vi "Dashboard Main.vi"() -> ()   [LabVIEW 2013]
uses:
  <vilib>/event_ctls.llb/eventvkey.ctl
  <vilib>/Rock Robotics/WPI/Dashboard/WPI_DashboardLogging Global.vi
  <vilib>/Utility/config.llb/Write Key (String).vi
  <vilib>/Utility/config.llb/Write Key (I32).vi
  <vilib>/Utility/config.llb/NI_LVConfig.lvlib
panel:
  out "Image Message":string="Timeout in Camera Communications"
  in  "Rec Mode":enum32{"Stop", "Record", "Playback"}(radio)
  in  "Dashboard Tab":T1(tab)
  out "Encoder Rate":dbl
  out "Encoder Count":dbl
  in  "Camera Settings":T2={"Frame Rate"=30, "Compression"=30, "Size"=1} {"Frame Rate" scale=1.0..30.0; "Size" items=["640x480", "320x240", "160x120"]}
  out "MotorSliders R":cluster{"MotorSlide1":dbl, "MotorSlide2":dbl} {"MotorSlide2" scale=-1.0..1.0 scale format="%#_2e"; "MotorSlide1" scale=-1.0..1.0 scale format="%#_2e"}
  out "MotorChart R":cluster{"Numeric":dbl, "Numeric":dbl}(graph)
  out "MotorSliders L":T3 {"MotorSlide4 2" scale=0.0..14.0 scale format="%#_2e"; "MotorSlide2" scale=-1.0..1.0 scale format="%#_2e"; "MotorSlide1" scale=-1.0..1.0 scale format="%#_2e"}
  out "MotorChart L":T4(graph)
  out "JS1 Z":dbl(slide) scale=-1.0..1.0 scale format="%#_2e"
  out "Joystick 1":cluster{"X":dbl, "Y":dbl}[](graph)
  out "JS Buttons 1":T5
  out "JS2 Z":dbl(slide) scale=-1.0..1.0 scale format="%#_2e"
  out "Joystick 2":cluster{"X":dbl, "Y":dbl}[](graph)
  out "JS Buttons 2":T5
  out "Mode":T6(ring)=enum."Auto Disabled"
  out "Camera IP":string
  in  "DB Camera Config":bool
  out "fps":dbl format="%#.1g"
  out "Mbps":dbl format="%#.1g"
  out "Mbps 2":bool
  out "LED 1":bool
  in  "Slider 1":dbl(slide) scale=0.0..100.0
  in  "Test Jag Num":u8
  in  "Test Jag Out":dbl min=-1.0 max=1.0
  in  "Checkbox 2":bool
  in  "Checkbox 1":bool
  in  "Test Slider":dbl(slide) scale=0.0..100.0 scale format="%#_3g"
  in  "On/Off":bool caption="Solenoid"
  in  "Test Name":u16(ring) items=["Select the test to run...", "Example Test", "-------------------------------", "List of tests is built in robot code.", "Replace with your own automated tests.", "Jag Test"]
  in  "Test Tree":string(tree)
  in  "Motor":cluster{"Value":dbl, "Enable":bool} {"Value" scale=-1.0..1.0 scale format="%#_3g"}
  out "Progress":T7 {"Test Progress" scale=0.0..100.0}
  in  "Rev/Fwd":cluster{"Forward":bool, "Reverse":bool}
  in  "Test Ring":u16(ring) items=["Auto", "Fixed indoor", "Fixed outdoor 1", "Fixed outdoor 2", "Fixed fluorescent 1", "Fixed fluorescent 2", "Hold current"]
  in  "Listbox":i32(listbox)
  out "Tree":string(tree)
  out "Camera Image":T8(plugin-control)
  in  "Enable":bool
  # "Left"
  # "Front"
  # "Right"
  # "Battery"
  # "Customize by placing controls and indicators here and name to\nmatch Dashboard Variables on robot."
  # "This tab is a great place for autonomous settings and validation.\nCustomize by placing controls and indicators here and name to\nmatch Dashboard Variables on robot."
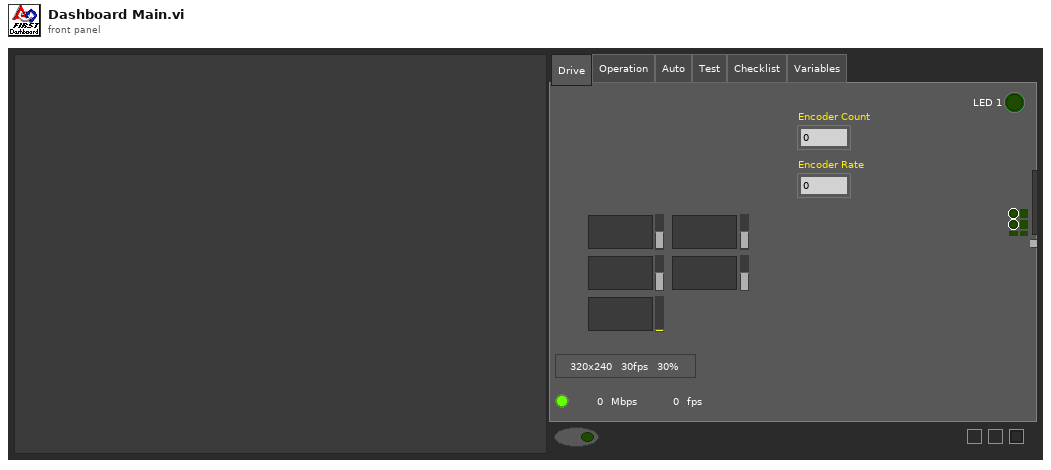
[diagram p1: front panel]
types:
  T1 = enum32{"Drive", "Operation", "Auto", "Test", "Checklist", "Variables"}
  T2 = cluster{"Frame Rate":i32, "Compression":i32, "Size":u16}
  T3 = cluster{"MotorSlide1":dbl, "MotorSlide2":dbl, "MotorSlide4 2":dbl}
  T4 = cluster{"Numeric":dbl, "Numeric":dbl, "Battery":sgl}
  T5 = cluster{bool, bool, bool, bool, bool, bool, bool, bool, bool, bool, bool, bool}
  T6 = enum8{"Tele-Op Disabled", "Tele-Op Enabled", "Auto Disabled", "Auto Enabled", "Test Disabled", "Test Enabled", ""}
  T7 = cluster{"Test Progress":u8, "Test Progress Text":string}
  T8 = typedef "IMAQ Image.ctl" = refnum<image>
  T9 = typedef "Image Type" = u32
  T10 = cluster{"Digital Inputs":bool[], "Digital Outputs":bool[]}
  T11 = cluster{"Competition mode":bool, "Robot Link":bool, "Autonomous":bool, "Enabled":bool, "E-Stop":bool, "Simulated":bool, "TestMode":bool, "Docked Window":bool}
  T12 = cluster{"Boolean Array[0]":bool, "Boolean Array[1]":bool, "Boolean Array[2]":bool, "Boolean Array[3]":bool, "Boolean Array[4]":bool, "Boolean Array[5]":bool, "Boolean Array[6]":bool, "Boolean Array[7]":bool, "Boolean Array[8]":bool, "Boolean Array[9]":bool, "Boolean Array[10]":bool, "Boolean Array[11]":bool}
  T13 = typedef "NI_LVConfig.lvlib/Config Data RefNum.ctl" = refnum<k1>
  T14 = typedef "eventvkey.ctl" = enum16{"ASCII", "Enter", "Return", "Shift", "Ctrl", "Alt", "Cmd", "Opt", "Caps", "NumLock", "Clear", "Break", "Up", "Down", "Left", "Right", "Insert", "Delete", "Home", "End", "PageUp", "PageDown", "Escape", "Help", "Pause", "ScrollLock", "F1", "F2", "F3", "F4", "F5", "F6", "F7", "F8", "F9", "F10", "F11", "F12", "F13", "F14", "F15", "F16", "F17", "F18", "F19", "F20", "F21", "F22", "F23", "F24", "Play", "VolumeUp", "VolumeDown", "Mute", "Two Byte Char"}
  T15 = cluster{"Image Size":bool, "Image Type":bool, "Pixel Value":bool, "ROI Information":bool, "Zoom Factor":bool}
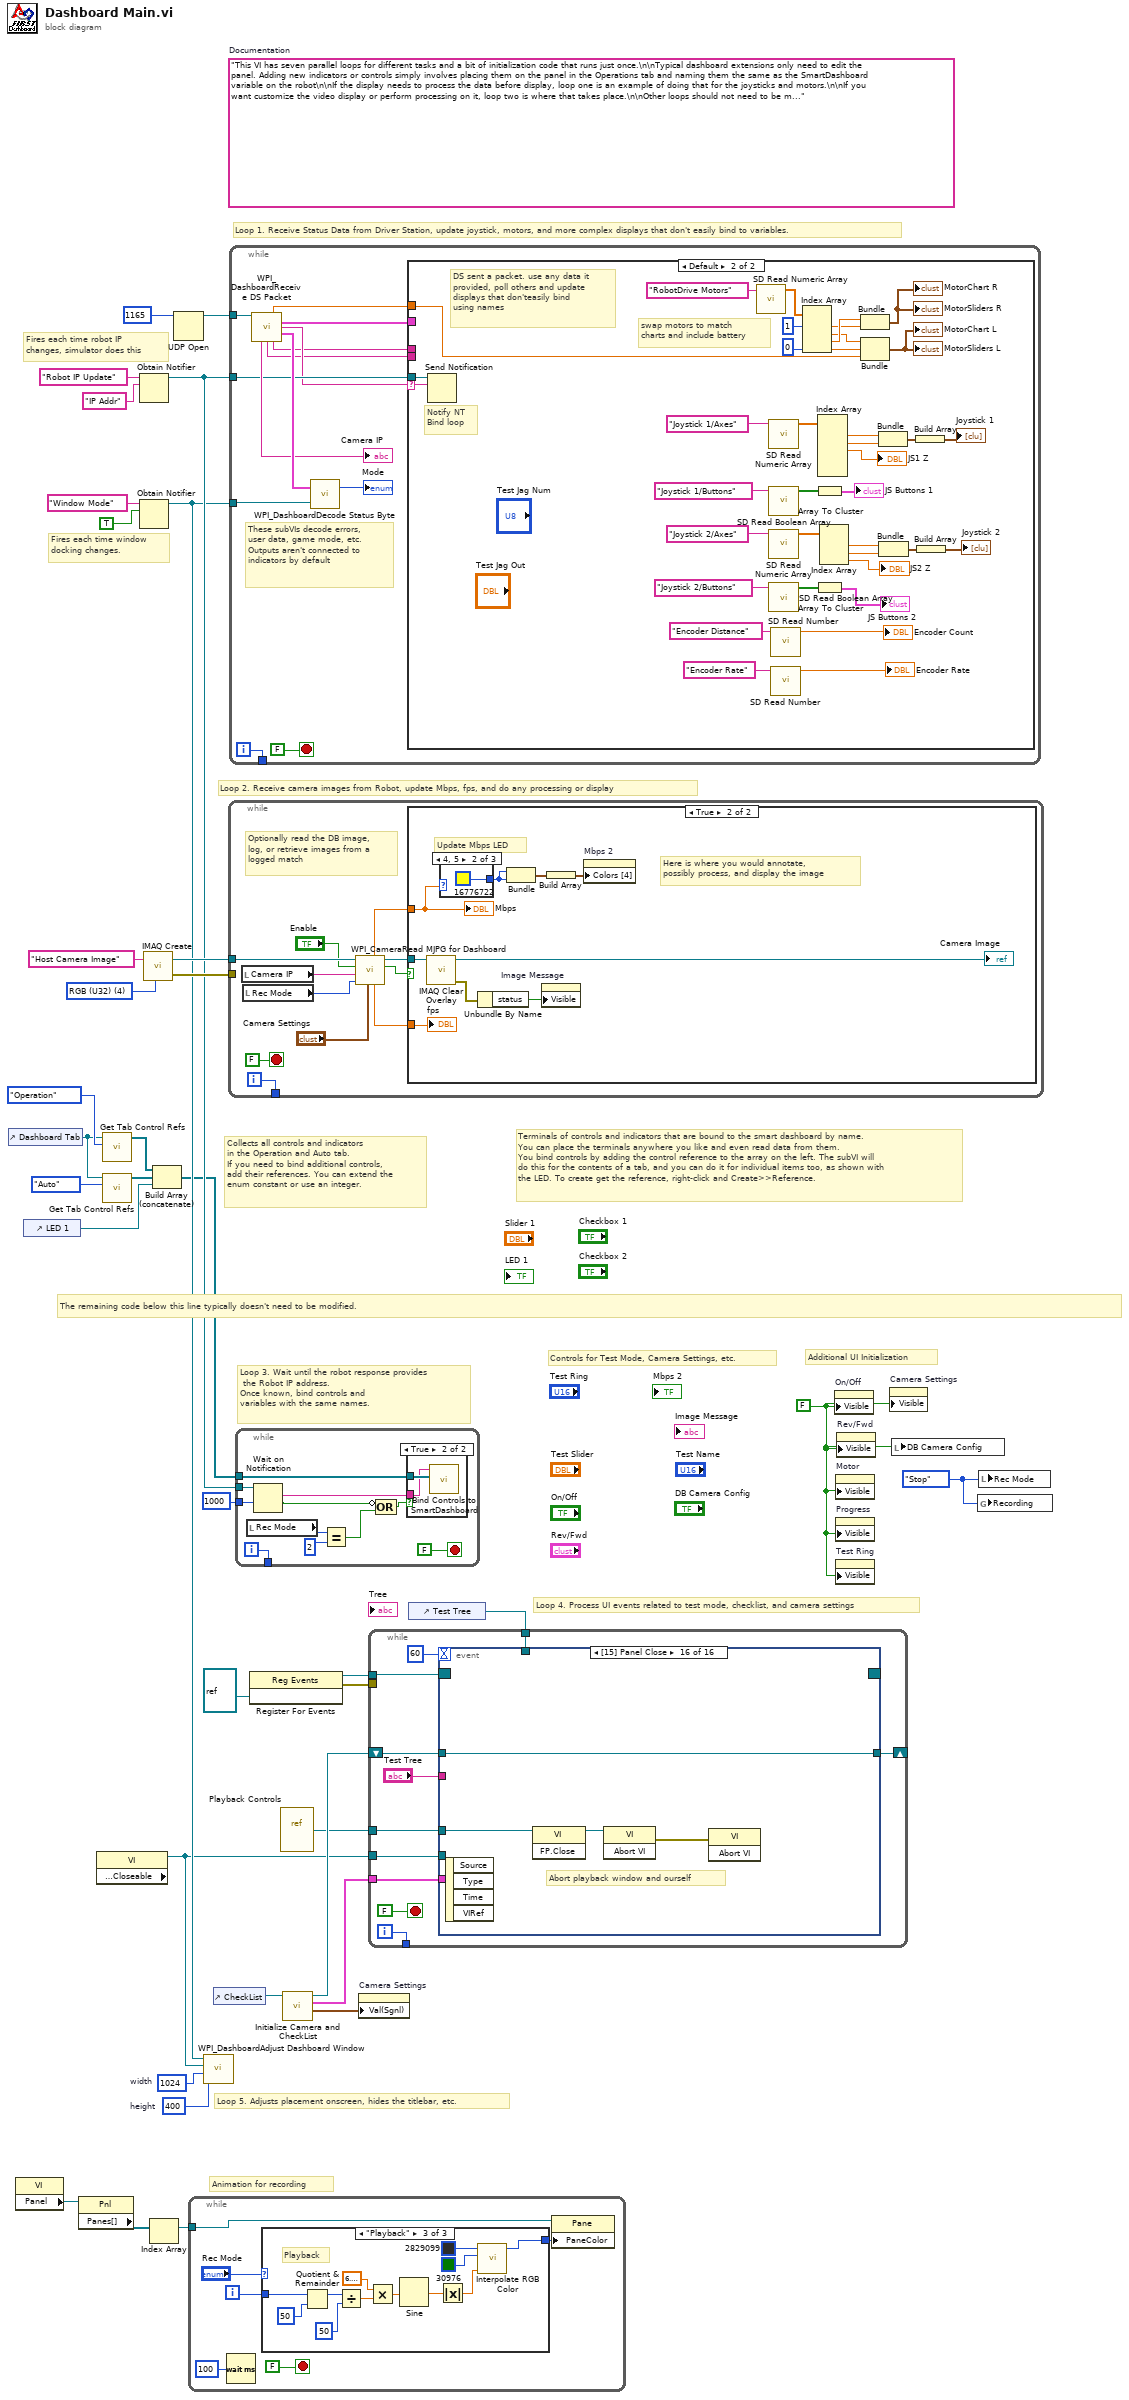
[diagram p0: block diagram]
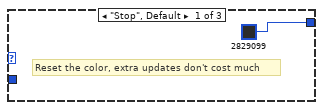
[diagram p2: hidden frame]
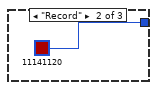
[diagram p3: hidden frame]
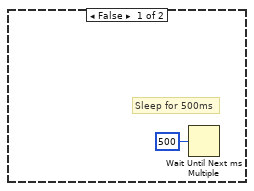
[diagram p5: hidden frame]
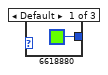
[diagram p6: hidden frame]
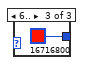
[diagram p7: hidden frame]
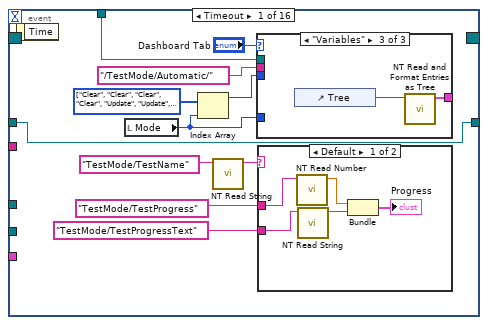
[diagram p8: hidden frame]
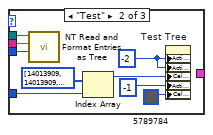
[diagram p10: hidden frame]
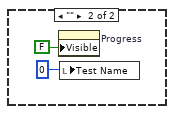
[diagram p11: hidden frame]
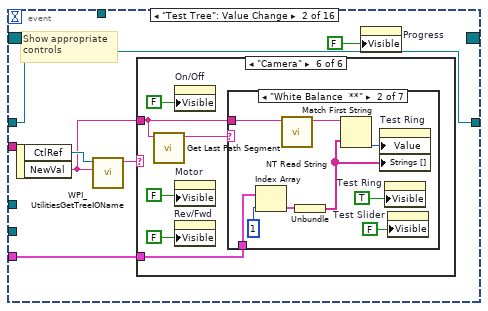
[diagram p12: hidden frame]
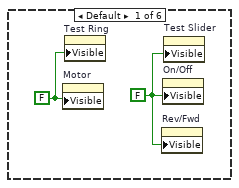
[diagram p13: hidden frame]
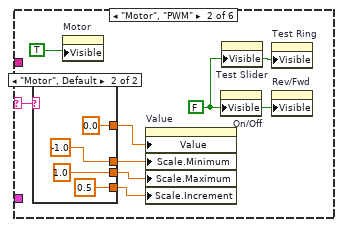
[diagram p14: hidden frame]
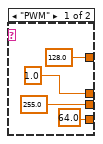
[diagram p15: hidden frame]
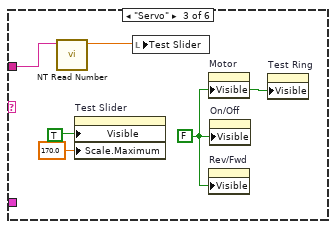
[diagram p16: hidden frame]
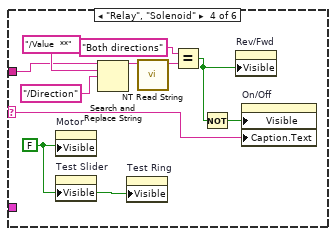
[diagram p17: hidden frame]
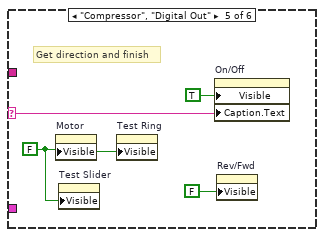
[diagram p18: hidden frame]
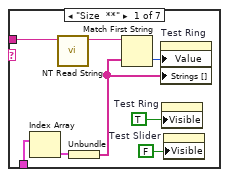
[diagram p19: hidden frame]
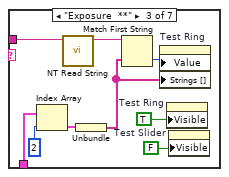
[diagram p20: hidden frame]
diagram:
  w8 = enum32{"Stop", "Record", "Playback"}."Stop" ("Rec Mode")
  w11 = 400  # height
  w12 = 1024  # width
  w25 = FALSE ("Visible")
  (unwired) "This VI has seven parallel loops for different tasks and a bit of initialization code that runs just once.\n\nTypical dashboard extensions only need to edit the panel. Adding new indicators or controls simply involves placing them on the panel in the Operations tab and naming them the same as the SmartDashboard variable on the robot\n\nIf the display needs to process the data before display, loop one is an example of doing that for the joysticks and motors.\n\nIf you want customize the video display or perform processing on it, loop two is where that takes place.\n\nOther loops should not need to be modified. They are pretty standard, and document the task they perform."  # Documentation
  w35 = T9 4 items=["Grayscale (U8)", "Grayscale (I16)", "Grayscale (SGL)", "Complex (CSG)", "RGB (U32)", "HSL (U32)", "RGB (U64)"] ("Image Type")
  # "Controls for Test Mode, Camera Settings, etc."
  # "Additional UI Initialization"
  # "Animation for recording"
  # "Fires each time robot IP\nchanges, simulator does this"
  # "Fires each time window\ndocking changes."
  # "Collects all controls and indicators\nin the Operation and Auto tab.\nIf you need to bind additional controls,\nadd their references. You can extend the\nenum constant or use an integer."
  # "The remaining code below this line typically doesn't need to be modified."
  # "Loop 4. Process UI events related to test mode, checklist, and camera settings"
  # "Terminals of controls and indicators that are bound to the smart dashboard by name.\nYou can place the terminals anywhere you like and even read data from them.\nYou bind controls by adding the control reference to the array on the left. The subVI will\ndo this for the contents of a tab, and you can do it for individual items too, as shown with\nthe LED. To create get the reference, right-click and Create>>Reference."
  # "Loop 3. Wait until the robot response provides\n the Robot IP address.\nOnce known, bind controls and\nvariables with the same names."
  # "Loop 5. Adjusts placement onscreen, hides the titlebar, etc."
  # "Loop 1. Receive Status Data from Driver Station, update joystick, motors, and more complex displays that don't easily bind to variables."
  # "Loop 2. Receive camera images from Robot, update Mbps, fps, and do any processing or display"
  n1 = control-ref of="Dashboard Tab"() -> (w6:refnum<vi>)
  n2 = property class="VI"() -> ("Panel"=w19:refnum<vi>)  [unwired: 2 in, 2 out]
  n3 = control-ref of="LED 1"() -> (w1:refnum<vi>)
  n4 = property class="Pnl"(reference=w19) -> ("Panes[]"=w20:refnum<vi>[])  [unwired: 1 in, 2 out]
  n5 = property class="VI" props=["Front Panel.Closeable"]() -> (reference out=w7:refnum<vi>)  [unwired: 2 in, 2 out]
  n6 = call <vilib>:"Get Tab Control Refs.vi"("Page Index"=T1."Operation" ("Dashboard Tab"), "TabControl in"=w6) -> ("ControlsOnPage"=w4:refnum<vi>[])  [unwired: 9 in]
  n7 = call <vilib>:"Get Tab Control Refs.vi"("Page Index"=T1."Auto" ("Dashboard Tab"), "TabControl in"=w6) -> ("ControlsOnPage"=w5:refnum<vi>[])  [unwired: 9 in]
  n8 = Obtain Notifier(name (unnamed)="Robot IP Update", notification data type="IP Addr" ("name (unnamed)")) -> (notifier out=w29:refnum<notifier>)  [unwired: 2 in, 2 out]
  n9 = Obtain Notifier(name (unnamed)="Window Mode", notification data type=TRUE) -> (notifier out=w10:refnum<notifier>)  [unwired: 2 in, 2 out]
  n10 = call "IMAQ Create"("Image Name"="Host Camera Image", "Image Type"=w35) -> ("New Image"=w33:T8, "error out"=w32:errorcluster)  [unwired: 2 in, 1 out]
  n11 = Index Array(array=w20) -> (element=w18:refnum<vi>)  [unwired: 1 in]
  n12 = Build Array (concatenate)(w4, w5, w1) -> (w3:refnum<vi>[])
  n13 = UDP Open(11:u16 1165 ("port")) -> (port=w36:refnum<k16>)  [unwired: 2 in, 4 out]
  n14 = while {
    tunnel: w18 -> [w39]
    i -> [w42]
    stop <- FALSE stop-if-true
    n15 = Wait (ms)(milliseconds to wait=u32 100) -> ()  [unwired: 1 out]
    n16 = case shown="\"Playback\"" "Rec Mode" {
      tunnel: w42 -> [_ _ w57]
      tunnel: [u32 2829099 ("Base Color") u32 11141120 ("Target Color") w46] -> w38
      frame "Stop", Default {
        # "Reset the color, extra updates don't cost much"
      }
      frame "Record" {
      }
      frame "Playback" {
        # "Playback"
        n17 = Quotient & Remainder(x=w57, y=u32 50 ("milliseconds to wait")) -> (x-y*floor(x/y)=w53:u32)  [unwired: 1 out]
        n18 = Divide(x=w53, y=u32 50 ("milliseconds to wait")) -> (x/y=w50:dbl)
        n19 = Multiply(x=6.283185307179586, y=w50) -> (x*y=w55:dbl)
        n20 = Sine(x=w55) -> (sin(x)=w54:dbl)
        n21 = Absolute Value(x=w54) -> (abs(x)=w47:dbl)
        n22 = call "Interpolate RGB Color.vi"("Proportion"=w47, "Target Color"=u32 30976, "Base Color"=u32 2829099) -> ("Result Color"=w46:u32)  [unwired: 8 in]
      }
    }
    n23 = property class="Pane"(reference=w39, "PaneColor"=w38) -> ()  [unwired: 1 in, 2 out]
  }
  n24 = call <vilib>:"WPI_DashboardAdjust Dashboard Window.vi"("height"=w11, "width"=w12, "reference in"=w7, "Notifier in"=w10) -> ()  [unwired: 8 in]
  n25 = control-ref of="CheckList"() -> (w9:refnum<vi>)
  n26 = while {
    tunnel: w33 -> [w66]
    tunnel: w32 -> [_]
    tunnel: [w67] -> _
    i -> [w67]
    stop <- FALSE stop-if-true
    # "Optionally read the DB image,\nlog, or retrieve images from a\nlogged match"
    n27 = local read "Camera IP"() -> (w59:string)
    n28 = local read "Rec Mode"() -> (w58:enum32{"Stop", "Record", "Playback"})
    n29 = call <vilib>:"WPI_CameraRead MJPG for Dashboard.vi"("Camera Settings"="Camera Settings", "Rec Mode"=w58, "Camera IP"=w59, "Enable"="Enable", "Refnum in"=w66) -> ("Active"=w63:bool, "Refnum out"=w65:T8, "FPS"=w62:dbl, "Bandwidth (Mbps)"=w61:dbl)  [unwired: 3 in]
    n30 = case shown="True" w63 {
      tunnel: w65 -> [_ w73]
      tunnel: w61 -> [_ w72]
      tunnel: w62 -> [_ w70]
      frame False {
        # "Sleep for 500ms"
        n31 = Wait Until Next ms Multiple(millisecond multiple=u32 500) -> ()  [unwired: 1 out]
      }
      frame True {
        # "Here is where you would annotate,\npossibly process, and display the image"
        # "Update Mbps LED"
        n32 = call "IMAQ Clear Overlay"("Image"=w73) -> ("error out"=w77:errorcluster, "Image Out"=→"Camera Image":T8)  [unwired: 2 in, 7 out]
        n33 = case shown="4, 5" w72 {
          tunnel: [u32 6618880 ("Color Box") u32 16776722 ("Color Box") u32 16716800 ("Color Box")] -> w74
          frame Default {
          }
          frame 4, 5 {
          }
          frame 6.. {
          }
        }
        n34 = Unbundle By Name(w77) -> ("status"=w78:bool)
        n35 = Bundle("Color Box"=w74, "Color Box"=w74) -> (w76:cluster{"Color Box":u32, "Color Box":u32})  [unwired: 1 out]
        n36 = property on="Image Message" class="Str"("Visible"=w78) -> ()  [unwired: 2 in, 2 out]
        n37 = Build Array(w76) -> (w75:cluster{"Color Box":u32, "Color Box":u32}[])
        n38 = property on="Mbps 2" class="Bool (strict)"("Colors [4]"=w75) -> ()  [unwired: 2 in, 2 out]
        "Mbps" <- w72
        "fps" <- w70
      }
    }
  }
  n39 = while {
    tunnel: w36 -> [w92]
    tunnel: w29 -> [w87]
    tunnel: w10 -> [w91]
    tunnel: [w88] -> _
    i -> [w88]
    stop <- FALSE stop-if-true
    # "These subVIs decode errors, user data, game mode, etc.\nOutputs aren't connected to indicators by default"
    n40 = call <vilib>:"WPI_DashboardReceive DS Packet.vi"("Recv Socket"=w92) -> ("Battery"=w82:sgl, "Driver Station"=w83:T10, "Robot IP Address"=w86:string, "Status"=w93:T11, "Camera IP Address"=→"Camera IP":string, "Low Priority User Data"=w85:string, "High Priority User Data"=w84:string)  [unwired: 1 in, 7 out]
    n41 = call <vilib>:"WPI_DashboardDecode Status Byte.vi"("Window Mode Notifier"=w91, "Status"=w93) -> ("Mode"=→"Mode":T6)  [unwired: 1 out]
    n42 = case shown="Default" w86 {
      selector: w86 -> [_ w109]
      tunnel: w87 -> [_ w110]
      tunnel: w85 -> [_ _]
      tunnel: w84 -> [_ _]
      tunnel: w83 -> [_ _]
      tunnel: w82 -> [_ w108]
      frame "0.0.0.0" {
        # "DS not sending packets, or no robot exists yet.\nDon't poll the variables"
      }
      frame Default {
        # "Notify NT\nBind loop"
        # "DS sent a packet. use any data it\nprovided, poll others and update\ndisplays that don'teasily bind\nusing names"
        # "swap motors to match\ncharts and include battery"
        n43 = Send Notification(notification=w109, notifier=w110) -> ()  [unwired: 1 in, 2 out]
        n44 = call <vilib>:"SD Read Numeric Array.vi"("Name"="RobotDrive Motors") -> ("Numeric Array"=w107:dbl[])  [unwired: 8 in, 2 out]
        n45 = call <vilib>:"SD Read Numeric Array.vi"("Name"="Joystick 1/Axes") -> ("Numeric Array"=w126:dbl[])  [unwired: 8 in, 2 out]
        n46 = call <vilib>:"SD Read Boolean Array.vi"("Name"="Joystick 1/Buttons") -> ("Boolean Array"=w128:bool[])  [unwired: 8 in, 2 out]
        n47 = call <vilib>:"SD Read Numeric Array.vi"("Name"="Joystick 2/Axes") -> ("Numeric Array"=w120:dbl[])  [unwired: 8 in, 2 out]
        n48 = call <vilib>:"SD Read Boolean Array.vi"("Name"="Joystick 2/Buttons") -> ("Boolean Array"=w119:bool[])  [unwired: 8 in, 2 out]
        n49 = call <vilib>:"SD Read Number.vi"("Name"="Encoder Distance") -> ("Numeric"=→"Encoder Count":dbl)  [unwired: 8 in, 2 out]
        n50 = call <vilib>:"SD Read Number.vi"("Name"="Encoder Rate") -> ("Numeric"=→"Encoder Rate":dbl)  [unwired: 8 in, 2 out]
        n51 = Index Array(array=w107, index #1=1, index #4=0) -> (element #1=w103:dbl, element #2=w102:dbl, element #3=w104:dbl, element #4=w99:dbl)  [unwired: 2 in]
        n52 = Array To Cluster(array=w128) -> (cluster=→"JS Buttons 1":T12)
        n53 = Array To Cluster(array=w119) -> (cluster=→"JS Buttons 2":T12)
        n54 = Index Array(array=w126) -> (element #1=w123:dbl, element #2=w124:dbl, element #3=→"JS1 Z":dbl)  [unwired: 6 in, 3 out]
        n55 = Index Array(array=w120) -> (element #1=w115:dbl, element #2=w114:dbl, element #3=→"JS2 Z":dbl)  [unwired: 3 in]
        n56 = Bundle("Numeric"=w104, "Numeric"=w103) -> (→"MotorChart R" →"MotorSliders R":cluster{"Numeric":dbl, "Numeric":dbl})  [unwired: 1 in]
        n57 = Bundle("Numeric"=w102, "Numeric"=w99, "Battery"=w108) -> (→"MotorChart L" →"MotorSliders L":T4)  [unwired: 1 in]
        n58 = Bundle("Numeric"=w123, "Numeric"=w124) -> (w122:cluster{"Numeric":dbl, "Numeric":dbl})  [unwired: 1 in]
        n59 = Bundle("Numeric"=w115, "Numeric"=w114) -> (w116:cluster{"Numeric":dbl, "Numeric":dbl})  [unwired: 1 in]
        n60 = Build Array(w122) -> (→"Joystick 1":cluster{"Numeric":dbl, "Numeric":dbl}[])
        n61 = Build Array(w116) -> (→"Joystick 2":cluster{"Numeric":dbl, "Numeric":dbl}[])
      }
    }
  }
  n62 = while {
    tunnel: w3 -> [w142]
    tunnel: w29 -> [w140]
    tunnel: [w138] -> _
    tunnel: u32 1000 ("milliseconds to wait") -> [w137]
    i -> [w138]
    stop <- FALSE stop-if-true
    n63 = local read "Rec Mode"() -> (w133:enum32{"Stop", "Record", "Playback"})
    n64 = Wait on Notification(notifier=w140, timeout in ms (-1)=w137) -> (notification=w139:string, timed out?=w135:bool)  [unwired: 2 in, 2 out]
    n65 = Equal?(x=w133, y=u16 2 ("Rec Mode")) -> (x = y?=w134:bool)
    n66 = Compound Arithmetic op=OR(invert w135, w134) -> (w136:bool)
    n67 = case shown="True" w136 {
      tunnel: w142 -> [_ w144]
      tunnel: w139 -> [_ w143]
      frame False {
      }
      frame True {
        n68 = call <vilib>:"Bind Controls to SmartDashboard.vi"("Bound Control Refs"=w144, "Server IP Address"=w143) -> ()  [unwired: 10 in]
      }
    }
  }
  n69 = register-events(refnum<vi> refnum) -> (reference out=w16:refnum<event-registration>, error out=w15:errorcluster)  [unwired: 2 in]
  n70 = vi-ref "Playback Controls.vi"() -> (w17:refnum<vi>)
  n71 = call "Initialize Camera and CheckList.vi"("ListBox in"=w9) -> ("Cluster"=w23:cluster{"value":i32, "value":i32, "index":i32}, "Array"=w24:cluster{string[]}[], "File Refnum"=w22:T13)  [unwired: 8 in]
  n72 = property on="Camera Settings" class="Clust (strict)"("Val(Sgnl)"=w23) -> ()  [unwired: 2 in, 2 out]
  n73 = control-ref of="Test Tree"() -> (w21:refnum<vi>)
  n74 = while {
    tunnel: w24 -> [w152]
    shift-right: [w151] -> _
    shift-left: w22 -> [w150]
    tunnel: [w149] -> _
    tunnel: w21 -> [w148]
    tunnel: w17 -> [w147]
    tunnel: w16 -> [w146]
    tunnel: w15 -> [_]
    tunnel: w7 -> [w145]
    i -> [w149]
    stop <- FALSE stop-if-true
    n75 = event shown="[15] Panel Close" {
      selector: w146 -> [_ _ _ _ _ _ _ _ _ _ _ _ _ _ _ _]
      dyn-events: [_ _ _ _ _ _ _ _ _ _ _ _ _ w390 _ _] -> _
      timeout: u32 60 ("milliseconds to wait") -> [_ _ _ _ _ _ _ _ _ _ _ _ _ _ _ _]
      tunnel: w148 -> [w162 _ _ _ _ _ _ _ _ _ _ _ _ _ _ _]
      tunnel: "Test Tree" -> [_ _ _ _ _ _ _ _ w359 w367 w369 w373 w381 _ _ _]
      tunnel: w152 -> [_ w186 _ _ _ _ w323 w353 _ _ _ _ _ _ _ _]
      tunnel: [w156 w185 w284 w289 w297 w309 w322 w346 w358 w365 w368 w372 w380 w392 w406 w407] -> w151
      tunnel: w150 -> [w156 w185 w284 w289 w297 w309 w321 w346 w358 w365 w368 w372 w380 w392 w406 w407]
      tunnel: w147 -> [_ _ _ _ _ _ _ _ _ _ _ _ _ w393 _ w410]
      tunnel: w145 -> [_ _ _ _ _ _ _ _ _ _ _ _ _ w388 _ _]
      event Timeout {
        w161 = enum16{"Update", "Clear"}[] [enum."Clear", enum."Clear", enum."Clear", enum."Clear", enum."Update", enum."Update", enum."Clear"] items=["Update", "Clear"]
        n76 = event-data() -> ()  [unwired: 1 in, 1 out]
        n77 = local read "Mode"() -> (w159:T6)
        n78 = Index Array(array=w161, index=w159) -> (element=w160:enum16{"Update", "Clear"})
        n79 = call <vilib>:"NT Read String.vi"("Name"="TestMode/TestName") -> ("String"=w165:string)  [unwired: 9 in, 1 out]
        n80 = case shown="\"Variables\"" "Dashboard Tab" {
          tunnel: w162 -> [_ w175 _]
          tunnel: "/TestMode/Automatic/" ("Name Pattern") -> [_ w174 _]
          tunnel: w160 -> [_ w173 _]
          tunnel: w159 -> [_ w171 _]
          tunnel: [_ _ w177] -> _
          frame "Operation", Default {
          }
          frame "Test" {
            w170 = -2 ("Active Item:Row Number")
            n81 = call <vilib>:"NT Read and Format Entries as Tree.vi"("Operation"=w173, "Name Pattern"=w174, "Tree Refnum"=w175) -> ()  [unwired: 7 in, 2 out]
            n82 = Index Array(array=u32[] [14013909, 14013909, 14013909, 14013909, 14013909, 16777215, 14013909], index=w171) -> (element=w169:u32)
            n83 = property on="Test Tree" class="Tree (strict)"("Active Item Row Number"=w170, "ActiveColNum"=w170, "CellBG"=w169, "Active Item Row Number"=-1 ("Active Item:Row Number"), "CellBG"=u32 5789784 ("Color Box")) -> ()  [unwired: 2 in, 2 out]
          }
          frame "Variables" {
            n84 = control-ref of="Tree"() -> (w176:refnum<vi>)
            n85 = call <vilib>:"NT Read and Format Entries as Tree.vi"("Tree Refnum"=w176) -> ("Formatted Strings"=w177:cluster{"Name":string, "Value":string}[])  [unwired: 9 in, 1 out]
          }
        }
        n86 = case shown="Default" w165 {
          tunnel: "TestMode/TestProgress" ("Name") -> [w179 _]
          tunnel: "TestMode/TestProgressText" ("Name") -> [w178 _]
          frame Default {
            n87 = call <vilib>:"NT Read Number.vi"("Name"=w179) -> ("Numeric"=w180:dbl)  [unwired: 9 in, 1 out]
            n88 = call <vilib>:"NT Read String.vi"("Name"=w178) -> ("String"=w181:string)  [unwired: 9 in, 1 out]
            n89 = Bundle("Numeric"=w180, "String"=w181) -> (→"Progress":cluster{"Numeric":dbl, "String":string})  [unwired: 1 in]
          }
          frame "" {
            n90 = property on="Progress" class="Clust (strict)"("Visible"=FALSE) -> ()  [unwired: 2 in, 2 out]
            n91 = local write "Test Name"(u16 0) -> ()
          }
        }
      }
      event "Test Tree": Value Change {
        # "Show appropriate\ncontrols"
        n92 = event-data() -> ("CtlRef"=w189:refnum<vi>, "NewVal"=w187:string)  [unwired: 1 in]
        n93 = call <vilib>:"WPI_UtilitiesGetTreeIOName.vi"("NewVal"=w187, "TreeControl in"=w189) -> ("I/O Name"=w190:string)  [unwired: 9 in]
        n94 = case shown="\"Camera\"" w190 {
          selector: w190 -> [_ w197 _ w215 w224 _]
          tunnel: w187 -> [_ _ w212 w214 _ w231]
          tunnel: w186 -> [_ _ _ _ _ w230]
          frame Default {
            w192 = FALSE ("Visible")
            w191 = FALSE ("Visible")
            n95 = property on="Motor" class="Clust (strict)"("Visible"=w191) -> ()  [unwired: 2 in, 2 out]
            n96 = property on="Test Ring" class="Ring (strict)"("Visible"=w191) -> ()  [unwired: 2 in, 2 out]
            n97 = property on="Rev/Fwd" class="Clust (strict)"("Visible"=w192) -> ()  [unwired: 2 in, 2 out]
            n98 = property on="On/Off" class="Bool (strict)"("Visible"=w192) -> ()  [unwired: 2 in, 2 out]
            n99 = property on="Test Slider" class="Slide (strict)"("Visible"=w192) -> ()  [unwired: 2 in, 2 out]
          }
          frame "Motor", "PWM" {
            w198 = FALSE ("Visible")
            n100 = case shown="\"Motor\", Default" w197 {
              tunnel: [1.0 ("Value") -1.0 ("Value")] -> w196
              tunnel: [255.0 ("Value") 1.0 ("Value")] -> w195
              tunnel: [128.0 ("Value") 0.0 ("Value")] -> w194
              tunnel: [64.0 ("Value") 0.5 ("Value")] -> w193
              frame "PWM" {
              }
              frame "Motor", Default {
              }
            }
            n101 = property on="Motor" class="Clust (strict)"("Visible"=TRUE) -> ()  [unwired: 2 in, 2 out]
            n102 = property on="Value" class="Slide (strict)"("Value"=w194, "Scale.Minimum"=w196, "Scale.Maximum"=w195, "Scale.Increment"=w193) -> ()  [unwired: 2 in, 2 out]
            n103 = property on="On/Off" class="Bool (strict)"("Visible"=w198) -> ()  [unwired: 2 in, 2 out]
            n104 = property on="Test Slider" class="Slide (strict)"("Visible"=w198) -> ()  [unwired: 2 in, 2 out]
            n105 = property on="Test Ring" class="Ring (strict)"("Visible"=w198) -> ()  [unwired: 2 in, 2 out]
            n106 = property on="Rev/Fwd" class="Clust (strict)"("Visible"=w198) -> ()  [unwired: 2 in, 2 out]
          }
          frame "Servo" {
            w210 = FALSE ("Visible")
            n107 = call <vilib>:"NT Read Number.vi"("Name"=w212) -> ("Numeric"=w211:dbl)  [unwired: 9 in, 1 out]
            n108 = property on="Test Slider" class="Slide (strict)"("Visible"=TRUE, "Scale.Maximum"=170.0 ("Scale.Range:Maximum")) -> ()  [unwired: 2 in, 2 out]
            n109 = local write "Test Slider"(w211) -> ()
            n110 = property on="Motor" class="Clust (strict)"("Visible"=w210) -> ()  [unwired: 2 in, 2 out]
            n111 = property on="Rev/Fwd" class="Clust (strict)"("Visible"=w210) -> ()  [unwired: 2 in, 2 out]
            n112 = property on="On/Off" class="Bool (strict)"("Visible"=w210) -> ()  [unwired: 2 in, 2 out]
            n113 = property on="Test Ring" class="Ring (strict)"("Visible"=w210) -> ()  [unwired: 2 in, 2 out]
          }
          frame "Relay", "Solenoid" {
            w213 = FALSE ("Visible")
            n114 = property on="Motor" class="Clust (strict)"("Visible"=w213) -> ()  [unwired: 2 in, 2 out]
            n115 = property on="Test Slider" class="Slide (strict)"("Visible"=w213) -> ()  [unwired: 2 in, 2 out]
            n116 = Search and Replace String(input string=w214, search string="/Value  **", replace string="/Direction") -> (result string=w220:string)  [unwired: 5 in, 3 out]
            n117 = property on="Test Ring" class="Ring (strict)"("Visible"=w213) -> ()  [unwired: 2 in, 2 out]
            n118 = call <vilib>:"NT Read String.vi"("Name"=w220) -> ("String"=w218:string)  [unwired: 9 in, 1 out]
            n119 = Equal?(x="Both directions", y=w218) -> (x = y?=w216:bool)
            n120 = Not(x=w216) -> (.not. x?=w217:bool)
            n121 = property on="Rev/Fwd" class="Clust (strict)"("Visible"=w216) -> ()  [unwired: 2 in, 2 out]
            n122 = property on="On/Off" class="Bool (strict)"("Visible"=w217, "Caption.Text"=w215) -> ()  [unwired: 2 in, 2 out]
          }
          frame "Compressor", "Digital Out" {
            w223 = FALSE ("Visible")
            # "Get direction and finish"
            n123 = property on="Motor" class="Clust (strict)"("Visible"=w223) -> ()  [unwired: 2 in, 2 out]
            n124 = property on="Test Slider" class="Slide (strict)"("Visible"=w223) -> ()  [unwired: 2 in, 2 out]
            n125 = property on="Test Ring" class="Ring (strict)"("Visible"=w223) -> ()  [unwired: 2 in, 2 out]
            n126 = property on="On/Off" class="Bool (strict)"("Visible"=TRUE, "Caption.Text"=w224) -> ()  [unwired: 2 in, 2 out]
            n127 = property on="Rev/Fwd" class="Clust (strict)"("Visible"=FALSE) -> ()  [unwired: 2 in, 2 out]
          }
          frame "Camera" {
            n128 = call <vilib>:"Get Last Path Segment.vi"("String in"=w231) -> ("String out"=w232:string)  [unwired: 10 in]
            n129 = property on="On/Off" class="Bool (strict)"("Visible"=FALSE) -> ()  [unwired: 2 in, 2 out]
            n130 = property on="Motor" class="Clust (strict)"("Visible"=FALSE) -> ()  [unwired: 2 in, 2 out]
            n131 = property on="Rev/Fwd" class="Clust (strict)"("Visible"=FALSE) -> ()  [unwired: 2 in, 2 out]
            n132 = case shown="\"White Balance  **\"" w232 {
              tunnel: w231 -> [w238 w247 w256 w265 w274 _ w280]
              tunnel: w230 -> [w236 w244 w253 w262 w271 _ _]
              frame "Size  **" {
                n133 = Index Array(array=w236) -> (element=w235:cluster{string[]})  [unwired: 1 in]
                n134 = call <vilib>:"NT Read String.vi"("Name"=w238) -> ("String"=w237:string)  [unwired: 9 in, 1 out]
                n135 = Unbundle(w235) -> (w233:string[])
                n136 = Match First String(2:w233, 3:w237) -> (0:w234:i32)  [unwired: 1 out]
                n137 = property on="Test Ring" class="Ring (strict)"("Value"=w234, "Strings []"=w233) -> ()  [unwired: 2 in, 2 out]
                n138 = property on="Test Ring" class="Ring (strict)"("Visible"=TRUE) -> ()  [unwired: 2 in, 2 out]
                n139 = property on="Test Slider" class="Slide (strict)"("Visible"=FALSE) -> ()  [unwired: 2 in, 2 out]
              }
              frame "White Balance  **" {
                n140 = Index Array(array=w244, index=1) -> (element=w245:cluster{string[]})
                n141 = call <vilib>:"NT Read String.vi"("Name"=w247) -> ("String"=w246:string)  [unwired: 9 in, 1 out]
                n142 = Unbundle(w245) -> (w242:string[])
                n143 = Match First String(2:w242, 3:w246) -> (0:w241:i32)  [unwired: 1 out]
                n144 = property on="Test Ring" class="Ring (strict)"("Value"=w241, "Strings []"=w242) -> ()  [unwired: 2 in, 2 out]
                n145 = property on="Test Ring" class="Ring (strict)"("Visible"=TRUE) -> ()  [unwired: 2 in, 2 out]
                n146 = property on="Test Slider" class="Slide (strict)"("Visible"=FALSE) -> ()  [unwired: 2 in, 2 out]
              }
              frame "Exposure  **" {
                n147 = Index Array(array=w253, index=2) -> (element=w254:cluster{string[]})
                n148 = call <vilib>:"NT Read String.vi"("Name"=w256) -> ("String"=w255:string)  [unwired: 9 in, 1 out]
                n149 = Unbundle(w254) -> (w250:string[])
                n150 = Match First String(2:w250, 3:w255) -> (0:w251:i32)  [unwired: 1 out]
                n151 = property on="Test Ring" class="Ring (strict)"("Value"=w251, "Strings []"=w250) -> ()  [unwired: 2 in, 2 out]
                n152 = property on="Test Ring" class="Ring (strict)"("Visible"=TRUE) -> ()  [unwired: 2 in, 2 out]
                n153 = property on="Test Slider" class="Slide (strict)"("Visible"=FALSE) -> ()  [unwired: 2 in, 2 out]
              }
              frame "Exposure Priority  **" {
                n154 = Index Array(array=w262, index=3) -> (element=w263:cluster{string[]})
                n155 = call <vilib>:"NT Read String.vi"("Name"=w265) -> ("String"=w264:string)  [unwired: 9 in, 1 out]
                n156 = Unbundle(w263) -> (w259:string[])
                n157 = Match First String(2:w259, 3:w264) -> (0:w260:i32)  [unwired: 1 out]
                n158 = property on="Test Ring" class="Ring (strict)"("Value"=w260, "Strings []"=w259) -> ()  [unwired: 2 in, 2 out]
                n159 = property on="Test Ring" class="Ring (strict)"("Visible"=TRUE) -> ()  [unwired: 2 in, 2 out]
                n160 = property on="Test Slider" class="Slide (strict)"("Visible"=FALSE) -> ()  [unwired: 2 in, 2 out]
              }
              frame "Color Enable  **" {
                n161 = Index Array(array=w271, index=4) -> (element=w272:cluster{string[]})
                n162 = call <vilib>:"NT Read String.vi"("Name"=w274) -> ("String"=w273:string)  [unwired: 9 in, 1 out]
                n163 = Unbundle(w272) -> (w268:string[])
                n164 = Match First String(2:w268, 3:w273) -> (0:w269:i32)  [unwired: 1 out]
                n165 = property on="Test Ring" class="Ring (strict)"("Value"=w269, "Strings []"=w268) -> ()  [unwired: 2 in, 2 out]
                n166 = property on="Test Ring" class="Ring (strict)"("Visible"=TRUE) -> ()  [unwired: 2 in, 2 out]
                n167 = property on="Test Slider" class="Slide (strict)"("Visible"=FALSE) -> ()  [unwired: 2 in, 2 out]
              }
              frame Default {
                n168 = property on="Test Ring" class="Ring (strict)"("Visible"=FALSE) -> ()  [unwired: 2 in, 2 out]
                n169 = property on="Test Slider" class="Slide (strict)"("Visible"=FALSE) -> ()  [unwired: 2 in, 2 out]
              }
              frame "Brightness  **", "Color Level  **", "Compression  **", "FPS  **", "Sharpness  **" {
                n170 = call <vilib>:"NT Read Number.vi"("Name"=w280) -> ("Numeric"=w279:dbl)  [unwired: 9 in, 1 out]
                n171 = local write "Test Slider"(w279) -> ()
                n172 = property on="Test Slider" class="Slide (strict)"("Visible"=TRUE, "Scale.Maximum"=100.0 ("Scale.Range:Maximum")) -> ()  [unwired: 2 in, 2 out]
                n173 = property on="Test Ring" class="Ring (strict)"("Visible"=FALSE) -> ()  [unwired: 2 in, 2 out]
              }
            }
          }
        }
        n174 = property on="Progress" class="Clust (strict)"("Visible"=FALSE) -> ()  [unwired: 2 in, 2 out]
      }
      event "Test Name": Mouse Enter {
        # "Populate the ring with the list of tests"
        n175 = event-data() -> ()  [unwired: 1 in, 1 out]
        n176 = call <vilib>:"NT Read String Array.vi"("Name"="TestMode/TestList") -> ("String Array"=w288:string[])  [unwired: 9 in, 1 out]
        n177 = Build Array (concatenate)("Select the test to run...", w288) -> (w287:string[])
        n178 = property on="Test Name" class="Ring (strict)"("Strings []"=w287) -> ()  [unwired: 2 in, 2 out]
      }
      event "Test Name": Value Change {
        w290 = FALSE ("Visible")
        # "Tell the robot the test name to run"
        n179 = event-data() -> ("NewVal"=w294:u16)  [unwired: 1 in]
        n180 = property on="Test Name" class="Ring (strict)"() -> ("Strings []"=w295:string[])  [unwired: 2 in, 2 out]
        n181 = local write "Progress"(T7 {"Test Progress"=0, "Test Progress Text"=""} ("Progress")) -> ()
        n182 = Index Array(array=w295, index=w294) -> (element=w293:string)
        n183 = call <vilib>:"NT Write String.vi"("String"=w293, "Name"="TestMode/TestName") -> ()  [unwired: 9 in, 1 out]
        n184 = property on="Progress" class="Clust (strict)"("Visible"=TRUE) -> ()  [unwired: 2 in, 2 out]
        n185 = property on="Motor" class="Clust (strict)"("Visible"=w290) -> ()  [unwired: 2 in, 2 out]
        n186 = property on="Test Slider" class="Slide (strict)"("Visible"=w290) -> ()  [unwired: 2 in, 2 out]
        n187 = property on="On/Off" class="Bool (strict)"("Visible"=w290) -> ()  [unwired: 2 in, 2 out]
        n188 = property on="Rev/Fwd" class="Clust (strict)"("Visible"=w290) -> ()  [unwired: 2 in, 2 out]
        n189 = property on="Test Ring" class="Ring (strict)"("Visible"=w290) -> ()  [unwired: 2 in, 2 out]
      }
      event "Listbox": Double Click {
        n190 = event-data() -> ("PlatMods.Shift"=w298:bool, "Row"=w300:i32)  [unwired: 1 in]
        n191 = case shown="True" w298 {
          tunnel: w300 -> [w304 _]
          tunnel: 1 -> [w303 _]
          frame False {
            n192 = property on="Listbox" class="LstBox (strict)"() -> ("Item Symbols"=w302:i32[])  [unwired: 2 in, 2 out]
            n193 = Replace Array Subset(array=w302, new element=w303, index=w304) -> (w301:i32[])
            n194 = property on="Listbox" class="LstBox (strict)"("Item Symbols"=w301) -> ()  [unwired: 2 in, 2 out]
          }
          frame True {
            w305 = 0 ("Top Row")
            n195 = property on="Listbox" class="LstBox (strict)"() -> ("Number of Rows"=w307:u32)  [unwired: 2 in, 2 out]
            n196 = Initialize Array(0, w307) -> (w306:i32[])
            n197 = property on="Listbox" class="LstBox (strict)"("Top Row"=w305, "Value"=w305, "Item Symbols"=w306) -> ()  [unwired: 2 in, 2 out]
          }
        }
      }
      event "Listbox": Key Down {
        n198 = event-data() -> ("VKey"=w311:T14)  [unwired: 1 in]
        n199 = case shown="\"Left\", \"Right\"" w311 {
          selector: w311 -> [w316 _]
          tunnel: eventvkey."Left" ("VKey") -> [w314 _]
          frame "Left", "Right" {
            n200 = Equal?(x=w314, y=w316) -> (x = y?=w315:bool)
            n201 = Select(t=0, s=w315, f=1) -> (s? t:f=w317:i32)
            n202 = property on="Listbox" class="LstBox (strict)"() -> ("Item Symbols"=w320:i32[])  [unwired: 2 in, 2 out]
            n203 = Replace Array Subset(array=w320, new element=w317, index="Listbox") -> (w319:i32[])
            n204 = property on="Listbox" class="LstBox (strict)"("Item Symbols"=w319) -> ()  [unwired: 2 in, 2 out]
          }
          frame Default {
          }
        }
      }
      event "DB Camera Config": Value Change {
        n205 = event-data() -> ("NewVal"=w324:bool)  [unwired: 1 in]
        n206 = case shown="False" w324 {
          tunnel: w323 -> [w333 _]
          tunnel: [w326 w344] -> w322
          tunnel: w321 -> [w325 w344]
          frame False {
            w340 = "Camera"
            w343 = FALSE ("Visible")
            n207 = local read "Camera Settings"() -> (w332:T2)
            n208 = Index Array(array=w333) -> (element=w336:cluster{string[]})  [unwired: 1 in]
            n209 = Unbundle(w332) -> ("Frame Rate"=w331:i32, "Compression"=w330:i32, "Size"=w334:u16)
            n210 = Unbundle(w336) -> (w335:string[])
            n211 = Index Array(array=w335, index=w334) -> (element=w329:string)
            n212 = call-poly <vilib>:"Write Key.vi"("section"=w340, "value"=w329, "key"="Size", "refnum"=w325) -> ("refnum out"=w342:T13)  [unwired: 2 in, 5 out]
            n213 = call-poly <vilib>:"Write Key.vi"("section"=w340, "value"=w331, "key"="FrameRate", "refnum"=w342) -> ("refnum out"=w341:T13)  [unwired: 1 in, 6 out]
            n214 = property on="Camera Settings" class="Clust (strict)"("Visible"=w343) -> ()  [unwired: 2 in, 2 out]
            n215 = local write "DB Camera Config"(w343) -> ()
            n216 = call-poly <vilib>:"Write Key.vi"("section"=w340, "value"=w330, "key"="Compression", "refnum"=w341) -> ("refnum out"=w327:T13)  [unwired: 1 in, 6 out]
            n217 = call <vilib>:"Close Config Data.vi"("refnum"=w327) -> ("file path"=w328:path)  [unwired: 2 in, 8 out]
            n218 = call <vilib>:"Open Config Data.vi"("configuration file path"=w328) -> ("refnum"=w326:T13)  [unwired: 8 in, 2 out]
          }
          frame True {
            n219 = property on="Camera Settings" class="Clust (strict)"("Visible"=TRUE) -> ()  [unwired: 2 in, 2 out]
          }
        }
      }
      event "Camera Settings": Value Change {
        n220 = event-data() -> ("NewVal"=w357:T2)  [unwired: 1 in]
        n221 = Index Array(array=w353) -> (element=w352:cluster{string[]})  [unwired: 1 in]
        n222 = Unbundle(w357) -> ("Frame Rate"=w348:i32, "Compression"=w347:i32, "Size"=w350:u16)
        n223 = Unbundle(w352) -> (w351:string[])
        n224 = Index Array(array=w351, index=w350) -> (element=w349:string)
        n225 = Format Into String(format string="%s   %dfps   %d%%", w349, w348, w347) -> (resulting string=w354:string)  [unwired: 2 in, 1 out]
        n226 = Build Array(w354) -> (w355:string[])
        n227 = property on="DB Camera Config" class="Bool (strict)"("Strings [4]"=w355) -> ()  [unwired: 2 in, 2 out]
      }
      event "Motor.Enable": Value Change {
        n228 = event-data() -> ("NewVal"=w363:bool)  [unwired: 1 in]
        n229 = Unbundle("Motor") -> ("Value"=w362:dbl)  [unwired: 1 out]
        n230 = Select(t=w362, s=w363, f=0.0) -> (s? t:f=w360:dbl)
        n231 = call <vilib>:"NT Write Number.vi"("Numeric"=w360, "Name"=w359) -> ()  [unwired: 9 in, 1 out]
      }
      event "Test Slider": Value Change {
        n232 = event-data() -> ("NewVal"=w366:dbl)  [unwired: 1 in]
        n233 = call <vilib>:"NT Write Number.vi"("Numeric"=w366, "Name"=w367) -> ()  [unwired: 9 in, 1 out]
      }
      event "On/Off": Value Change {
        n234 = event-data() -> ("NewVal"=w371:bool)  [unwired: 1 in]
        n235 = Boolean To (0,1)(Boolean=w371) -> (0, 1=w370:i16)
        n236 = call <vilib>:"NT Write Number.vi"("Numeric"=w370, "Name"=w369) -> ()  [unwired: 9 in, 1 out]
      }
      event "Rev/Fwd": Value Change {
        n237 = event-data() -> ("NewVal.Forward"=w379:bool, "NewVal.Reverse"=w378:bool)  [unwired: 1 in]
        n238 = Boolean To (0,1)(Boolean=w379) -> (0, 1=w375:i16)
        n239 = Boolean To (0,1)(Boolean=w378) -> (0, 1=w377:i16)
        n240 = Negate(x=w377) -> (-x=w376:i16)
        n241 = Add(x=w375, y=w376) -> (x+y=w374:i16)
        n242 = call <vilib>:"NT Write Number.vi"("Numeric"=w374, "Name"=w373) -> ()  [unwired: 9 in, 1 out]
      }
      event "Test Ring": Value Change {
        n243 = event-data() -> ("NewVal"=w383:u16)  [unwired: 1 in]
        n244 = property on="Test Ring" class="Ring (strict)"() -> ("Strings []"=w384:string[])  [unwired: 2 in, 2 out]
        n245 = Index Array(array=w384, index=w383) -> (element=w382:string)
        n246 = call <vilib>:"NT Write String.vi"("String"=w382, "Name"=w381) -> ()  [unwired: 9 in, 1 out]
      }
      event "Rec Mode": Value Change {
        # "Update globals for recording mode and path to read log from.\nClear when logging and let NetworkTables set path for vision to\nuse."
        n247 = event-data() -> ("NewVal"=w394:enum32{"Stop", "Record", "Playback"})  [unwired: 1 in]
        n248 = global write "WPI_DashboardLogging Global.vi" "Logging Filename"(path "") -> ()
        n249 = case shown="\"Stop\", \"Record\"" w394 {
          tunnel: w393 -> [_ w396 w404]
          tunnel: [_ _ w403] -> w390
          tunnel: [_ _ w402] -> _
          tunnel: w388 -> [_ _ w400]
          tunnel: cluster{i32, i32} {-250, 170} -> [_ _ w399]
          tunnel: [_ _ T15 {"Image Size"=TRUE, "Image Type"=TRUE, "Pixel Value"=TRUE, "ROI Information"=TRUE, "Zoom Factor"=FALSE} ("Image Information Shown:All Elements")] -> w386
          tunnel: [_ _ TRUE ("Zoom Factor")] -> w385
          frame Default {
          }
          frame "Stop", "Record" {
            # "Place Window too"
            n250 = invoke class="VI" method="FP.Close"(reference=w396) -> (reference out=w395:refnum<vi>)  [unwired: 2 in, 2 out]
            n251 = invoke class="VI" method="Abort VI"(reference=w395) -> ()  [unwired: 2 in, 3 out]
          }
          frame "Playback" {
            n252 = call "Open Playback Panel.vi"("Offset"=w399, "DB VI Ref"=w400, "Playback in"=w404) -> ("Playback out"=w401:refnum<vi>)  [unwired: 8 in]
            n253 = register-events(w401) -> (reference out=w403:refnum<event-registration>, error out=w402:errorcluster)  [unwired: 2 in]
          }
        }
        n254 = global write "WPI_DashboardLogging Global.vi" "Recording"(w394) -> ()
        n255 = property on="Camera Image" class="ImageControl"("Image Information Shown"=w386, "Image Information Visible"=w385) -> ()  [unwired: 2 in, 2 out]
        n256 = call <vilib>:"WPI_DashboardNT Log FieldName Cache.vi"("Operation"=enum16{"Lookup/Add", "Index", "Clear"}."Clear") -> ()  [unwired: 8 in, 3 out]
      }
      event Panel Close {
        w405 = enum32{"Stop", "Record", "Playback"}."Stop" ("Rec Mode")
        n257 = event-data() -> ()  [unwired: 1 in, 4 out]
        n258 = local write "Rec Mode"(w405) -> ()
        n259 = global write "WPI_DashboardLogging Global.vi" "Recording"(w405) -> ()
      }
      event Panel Close {
        # "Abort playback window and ourself"
        n260 = event-data() -> ()  [unwired: 1 in, 4 out]
        n261 = invoke class="VI" method="FP.Close"(reference=w410) -> (reference out=w409:refnum<vi>)  [unwired: 2 in, 2 out]
        n262 = invoke class="VI" method="Abort VI"(reference=w409) -> (error out=w408:errorcluster)  [unwired: 2 in, 2 out]
        n263 = invoke class="VI" method="Abort VI"(error in=w408) -> ()  [unwired: 2 in, 3 out]
      }
    }
  }
  n264 = property on="On/Off" class="Bool (strict)"("Visible"=w25) -> ()  [unwired: 2 in, 2 out]
  n265 = property on="Motor" class="Clust (strict)"("Visible"=w25) -> ()  [unwired: 2 in, 2 out]
  n266 = property on="Progress" class="Clust (strict)"("Visible"=w25) -> ()  [unwired: 2 in, 2 out]
  n267 = property on="Test Ring" class="Ring (strict)"("Visible"=w25) -> ()  [unwired: 2 in, 2 out]
  n268 = property on="Rev/Fwd" class="Clust (strict)"("Visible"=w25) -> ()  [unwired: 2 in, 2 out]
  n269 = property on="Camera Settings" class="Clust (strict)"("Visible"=w25) -> ()  [unwired: 2 in, 2 out]
  n270 = local write "DB Camera Config"(w25) -> ()
  n271 = global write "WPI_DashboardLogging Global.vi" "Recording"(w8) -> ()
  n272 = local write "Rec Mode"(w8) -> ()
